vi "CheckInOpened.vi"(8 "error in (no error)":errorcluster, 10 "GUID":string, 11 "SMO.UI.MAUI in":refnum<class "SMO.UI.MAUI.lvclass">) -> (0 "error out":errorcluster, 1 "Index":i32, 2 "InOpened?":bool, 3 "SMO.UI.MAUI out":refnum<class "SMO.UI.MAUI.lvclass">)   [LabVIEW 2020, in "SMO.UI.MAUI.lvclass"]
uses:
  SMO.UI.MAUI.lvclass
  SMO.UI.MAUI.lvclass/SMO.UI.MAUI.ctl
  <vilib>/Levylab/SMO.UI.Embedded/SMO.UI.Embedded.lvclass
  C:/Program Files (x86)/National Instruments/LabVIEW 2020/vi.lib/JKI/JKI SMO/SMO/SMO.lvclass
  <vilib>/JKI/JKI SMO/SMO/SMO.lvclass
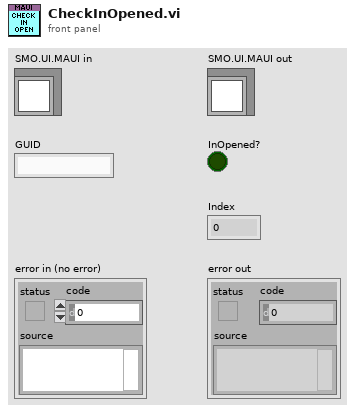
[diagram p1: front panel]
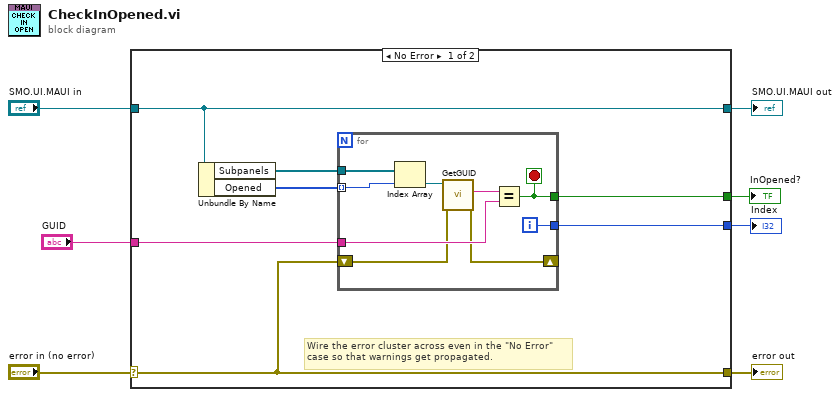
[diagram p0: block diagram]
diagram:
  n1 = case shown="No Error" "error in (no error)" {
    selector: "error in (no error)" -> [w10 w25]
    tunnel: [w10 w25] -> w6
    tunnel: [w14 w24] -> w4
    tunnel: "SMO.UI.MAUI in" -> [w14 w24]
    tunnel: "GUID" -> [w11 _]
    tunnel: [w9 _] -> w2
    tunnel: [w8 _] -> w1
    frame No Error {
      # "Wire the error cluster across even in the \"No Error\"\ncase so that warnings get propagated."
      n2 = Unbundle By Name(w14) -> ("Subpanels"=w13:refnum<class "SMO.UI.Embedded.lvclass">[], "Opened"=w12:i32[])
      n3 = for {
        tunnel: w13 -> [w23]
        tunnel: w12 -> [w16] mode=indexing
        tunnel: w11 -> [w20]
        shift-right: [w18] -> _
        shift-left: w10 -> [w19]
        tunnel: [w17] -> w9
        tunnel: [w15] -> w8
        i -> [w15]
        stop <- w17 stop-if-true
        n4 = Index Array(array=w23, index=w16) -> (element=w22:refnum<class "SMO.UI.Embedded.lvclass">)
        n5 = call <vilib>:"GetGUID.vi"("error in (no error)"=w19, "SMO"=w22) -> ("error out"=w18:errorcluster, "GUID"=w21:string)  [unwired: 7 in, 1 out]
        n6 = Equal?(x=w21, y=w20) -> (x = y?=w17:bool)
      }
    }
    frame Error {
    }
  }
  "error out" <- w6
  "SMO.UI.MAUI out" <- w4
  "InOpened?" <- w2
  "Index" <- w1
